vi "CBOR to JSON.vi"(8 "error in (no error)":errorcluster, 11 "CBOR Hex":string) -> (3 "JSON Object":string)   [LabVIEW 2020, in "CBOR.lvlib"]
doc: "Convert JSON object into CBOR Hex."
uses:
  CBOR.lvlib
panel:
  out "error out":errorcluster
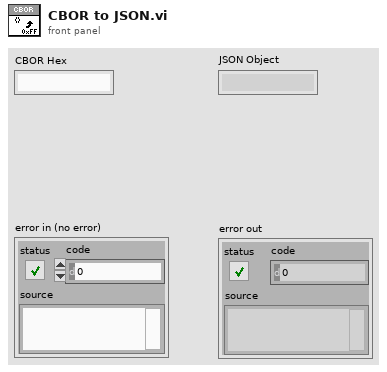
[diagram p1: front panel]
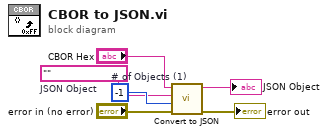
[diagram p0: block diagram]
diagram:
  w1 = ""  # JSON Object
  w2 = -1  # # of Objects (1)
  n1 = call "Convert to JSON.vi"("error in (no error)"="error in (no error)", "# of Objects (-1 : All)"=w2, "JSON Object (empty)"=w1, "CBOR Hex"="CBOR Hex") -> ("error out"=→"error out":errorcluster, "<JSON Object>"=→"JSON Object":string)  [unwired: 5 in, 1 out]
